vi "SpreadsheetStorage.vi"() -> ()   [LabVIEW 2015]
uses:
  <vilib>/Utility/file.llb/Write Delimited Spreadsheet (DBL).vi
panel:
  in  "Waveform Parameters":cluster{"Frequency":dbl, "Amplitude":dbl}
  in  "Digitizing Parameters":T1
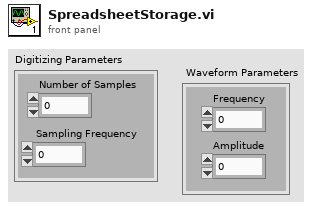
[diagram p1: front panel]
types:
  T1 = cluster{"Number of Samples":dbl, " Sampling Frequency":dbl}
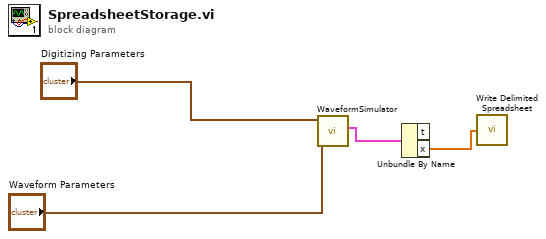
[diagram p0: block diagram]
diagram:
  n1 = call "WaveformSimulator.vi"("Waveform Parameters"="Waveform Parameters", "Digitizing Parameters"="Digitizing Parameters") -> ("XY Graph"=w2:cluster{"t":dbl[], "x":dbl[]})  [unwired: 9 in]
  n2 = Unbundle By Name(w2) -> ("x"=w1:dbl[])  [unwired: 1 out]
  n3 = call-poly <vilib>:"Write Delimited Spreadsheet.vi"("1D data"=w1) -> ()  [unwired: 13 in, 2 out]
